vi "Destroy.vi"(8 "error in (no error)":errorcluster, 11 "Dictionary in":refnum<class "Dictionary.lvclass">) -> (0 "error out":errorcluster, 1 "Values":variant[](array[variant]), 2 "Keys":string[](array[string]))   [LabVIEW 2018, in "Application.lvlib" / "Dictionary.lvclass"]
uses:
  Dictionary.lvclass
  Dictionary.lvclass/Dictionary.ctl
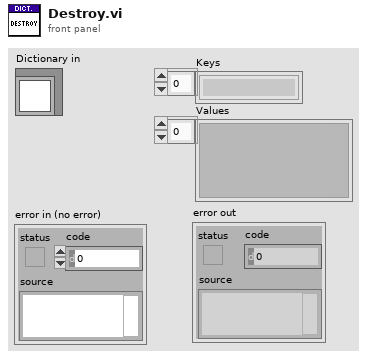
[diagram p1: front panel]
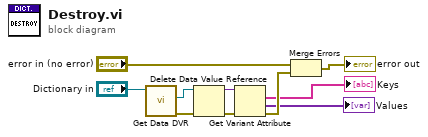
[diagram p0: block diagram]
diagram:
  n1 = call "Get Data DVR.vi"("Dictionary in"="Dictionary in") -> ("error out"=w7:errorcluster, "Data DVR"=w8:refnum<data-value>)  [unwired: 8 in, 1 out]
  n2 = Delete Data Value Reference(data value reference=w8, error in=w7) -> (data value=w3:variant, error out=w4:errorcluster)
  n3 = Get Variant Attribute(Variant=w3, error in=w4) -> (names=→"Keys":string[], values=→"Values":variant[], error out=w10:errorcluster)  [unwired: 2 in, 1 out]
  n4 = Merge Errors("error in (no error)", w10) -> (→"error out":errorcluster)
